vi "探头窗口-20-网络版.vi"() -> ()   [LabVIEW 2017]
panel:
  in  "外部停止命令？":bool=TRUE
  out "引用-监测模式？":refnum<vi>
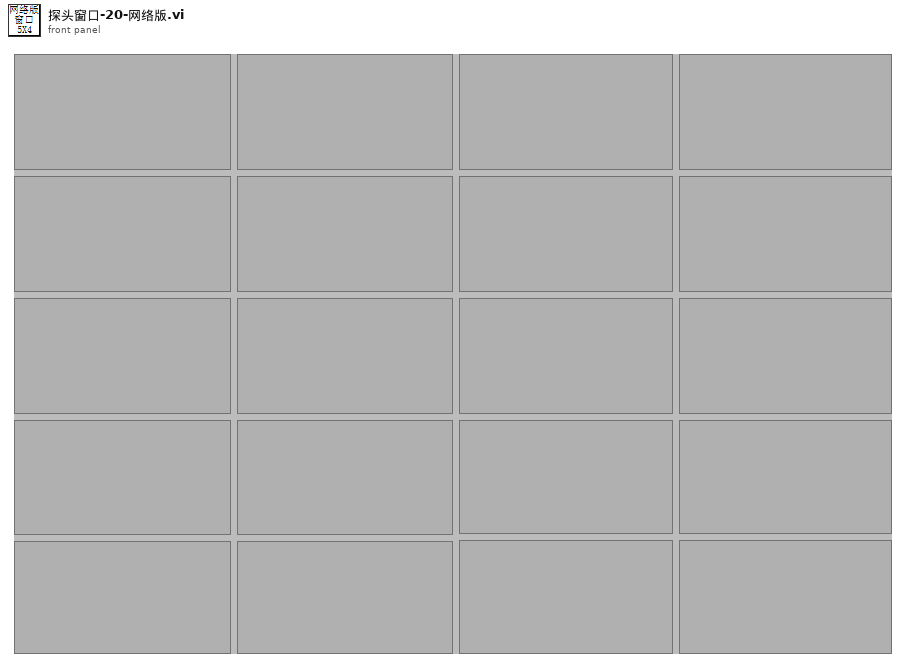
[diagram p1: front panel]
types:
  T1 = typedef "eventvkey.ctl" = enum16{"ASCII", "Enter", "Return", "Shift", "Ctrl", "Alt", "Cmd", "Opt", "Caps", "NumLock", "Clear", "Break", "Up", "Down", "Left", "Right", "Insert", "Delete", "Home", "End", "PageUp", "PageDown", "Escape", "Help", "Pause", "ScrollLock", "F1", "F2", "F3", "F4", "F5", "F6", "F7", "F8", "F9", "F10", "F11", "F12", "F13", "F14", "F15", "F16", "F17", "F18", "F19", "F20", "F21", "F22", "F23", "F24", "Play", "VolumeUp", "VolumeDown", "Mute", "Two Byte Char"}
  T2 = typedef "探头属性.ctl" = cluster{"探头地址与信息":T3, "测量值":T6, "限值":T7, "探头状态":T8, "累积记录":T9, "报警方式":T10}
  T3 = typedef "探测器信息.ctl" = cluster{"网络地址":string, "名称":string, "备注":string, "累积剂量":dbl, "累积限值":dbl, "硬件剂量率限值":T4, "剂量率限值1":dbl, "剂量率限值2":dbl, "报警方式":T5}
  T4 = typedef "探头剂量率限值选择.ctl" = enum16{"一级限值", "二级限值"}
  T5 = typedef "报警方式选择.ctl" = enum16{"常报警", "自动静音", "手动静音"}
  T6 = typedef "测量值.ctl" = cluster{"时间":timestamp, "数值":dbl}
  T7 = typedef "剂量率限值.ctl" = cluster{"限值1":dbl, "限值2":dbl, "探头限值":T4}
  T8 = typedef "探头状态.ctl" = enum16{"正常", "离线", "禁用", "一级报警", "二级报警", "累积报警"}
  T9 = typedef "单条累积记录.ctl" = cluster{"起始时间":timestamp, "结束时间":timestamp, "累积剂量":dbl}
  T10 = typedef "报警方式.ctl" = cluster{"报警方式":T5, "延迟计时":u16, "报警中？":bool}
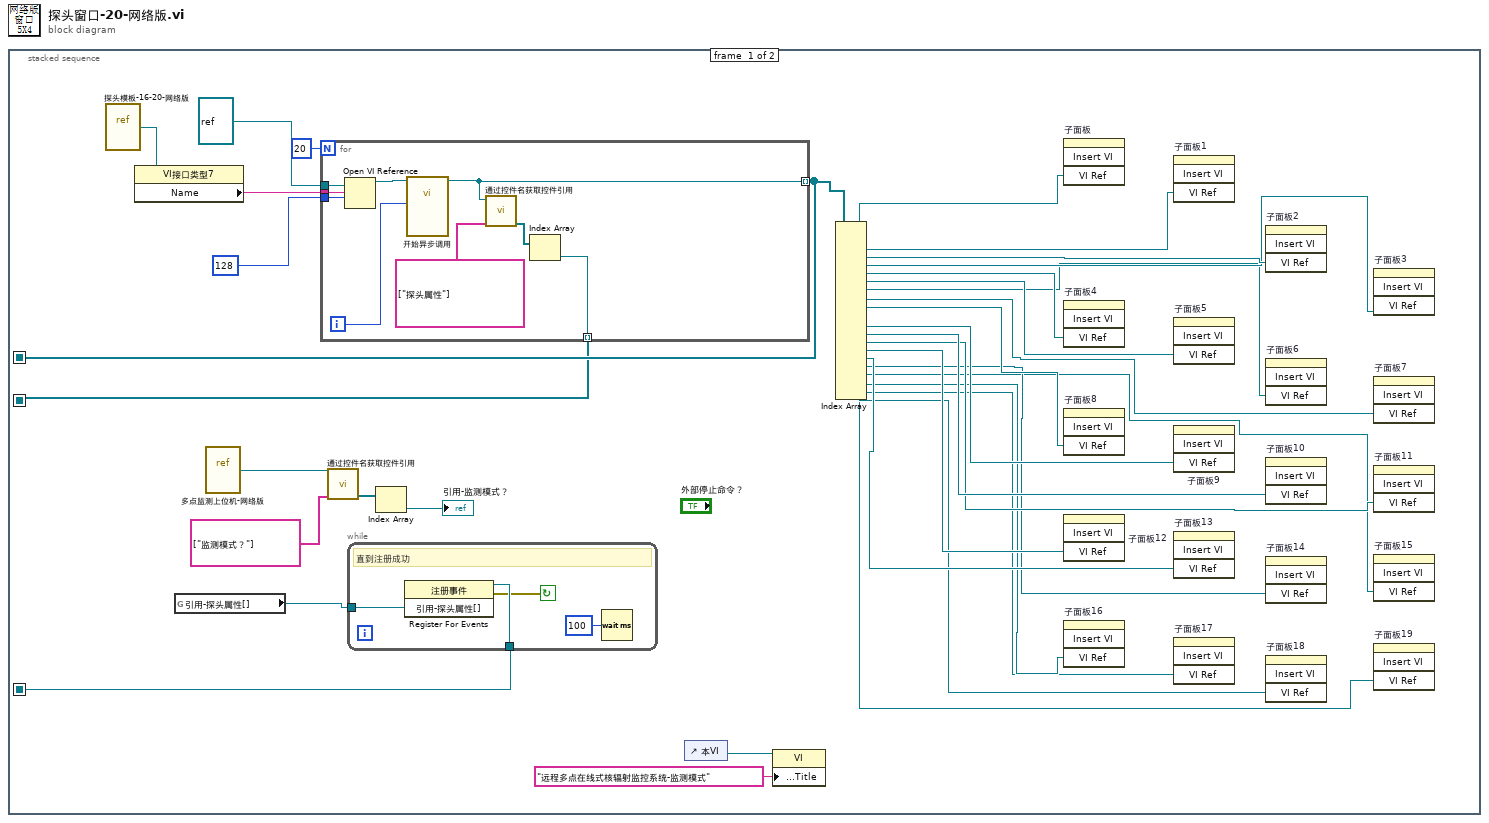
[diagram p0: block diagram]
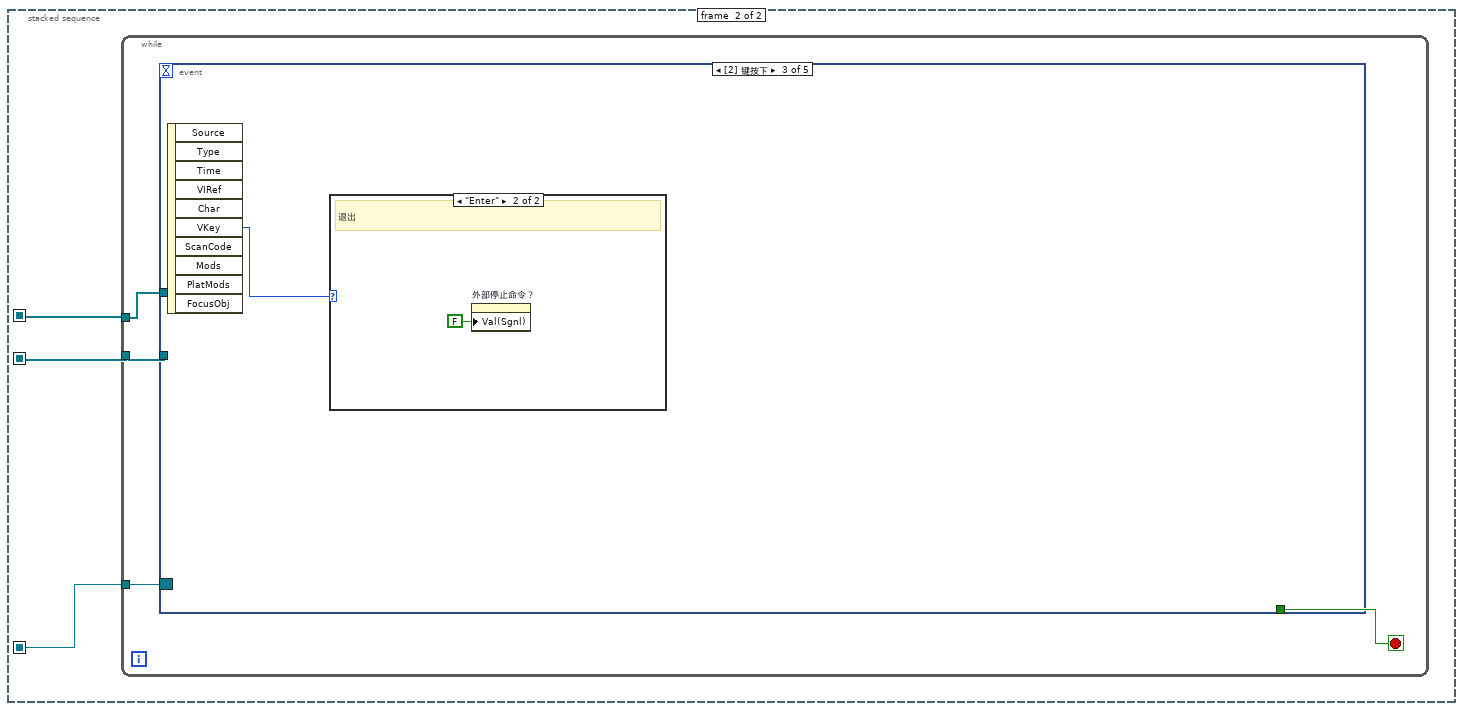
[diagram p2: hidden frame]
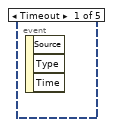
[diagram p3: hidden frame]
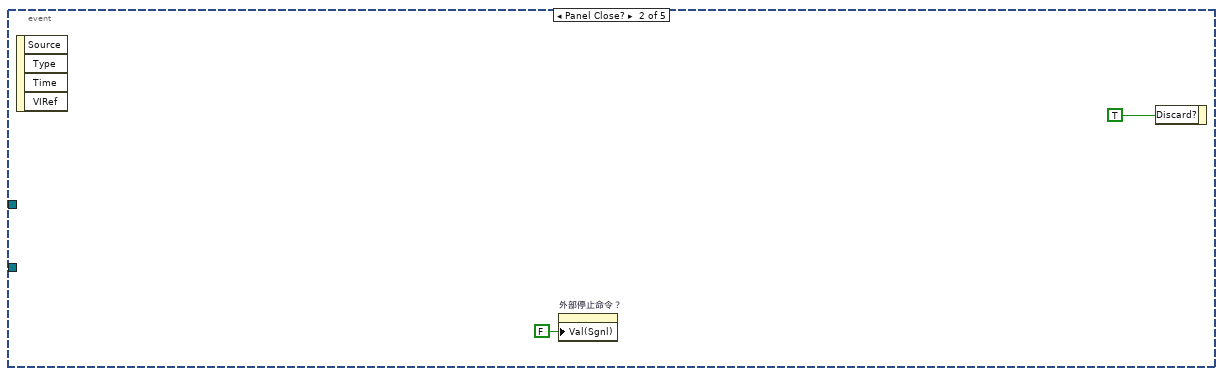
[diagram p4: hidden frame]
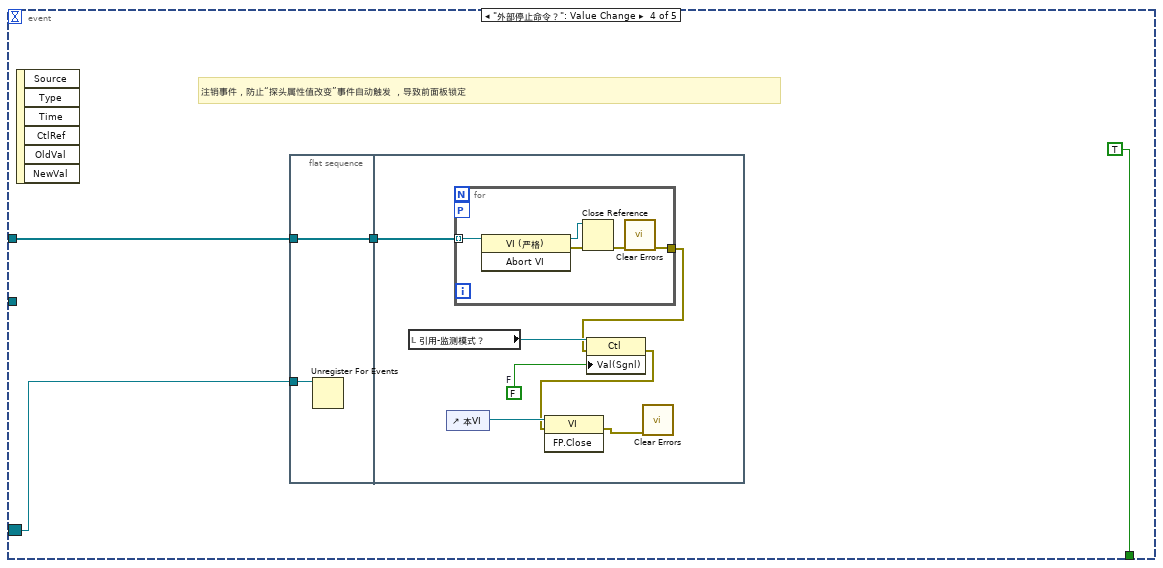
[diagram p6: hidden frame]
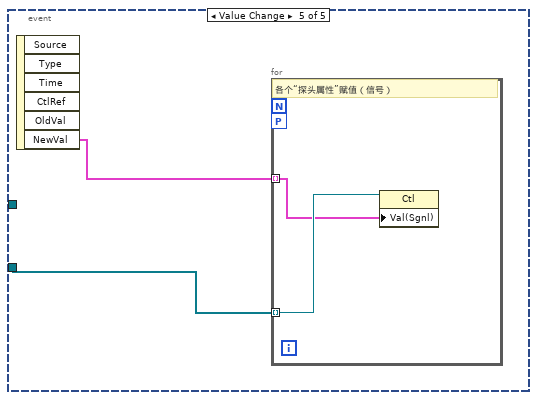
[diagram p7: hidden frame]
diagram:
  n1 = stacked-sequence {
    seq-local: [w30 _] -> [_ w51]
    seq-local: [w9 _] -> [_ w50]
    seq-local: [w1 _] -> [_ w49]
    frame #0 {
      n2 = vi-ref "探头模板-16-20-网络版.vi"() -> (w35:refnum<vi>)
      n3 = property class="VI接口类型7"(reference=w35) -> ("Name"=w34:string)  [unwired: 1 in, 2 out]
      n4 = global read "全局变量-35点监测.vi" "引用-探头属性[]"() -> (w2:refnum<vi>)
      n5 = vi-ref "多点监测上位机-网络版.vi"() -> (w5:refnum<vi>)
      n6 = for {
        N: 20 -> [_]
        tunnel: w34 -> [w48]
        tunnel: 128 ("选项") -> [w47]
        tunnel: refnum<vi> refnum ("类型说明符VI引用句柄（仅用于类型）") -> [w46]
        tunnel: [w41] -> w30 mode=indexing
        tunnel: [w42] -> w9 mode=indexing
        i -> [w40]
        n7 = Open VI Reference(type specifier VI Refnum (for type only)=w46, vi path=w48, options=w47) -> (vi reference=w43:refnum<vi>)  [unwired: 3 in, 1 out]
        n8 = call-by-ref "开始异步调用"(reference=w43, "探头序号"=w40) -> (reference out=w41:refnum<vi>)  [unwired: 12 in, 1 out]
        n9 = call "通过控件名获取控件引用.vi"("控件名数组"=string[] ["探头属性"], "VI引用"=w41) -> ("控件引用输出"=w45:refnum<vi>[])  [unwired: 7 in, 2 out]
        n10 = Index Array(array=w45) -> (element=w42:refnum<vi>)  [unwired: 1 in]
      }
      n11 = call "通过控件名获取控件引用.vi"("控件名数组"=string[] ["监测模式？"], "VI引用"=w5) -> ("控件引用输出"=w7:refnum<vi>[])  [unwired: 7 in, 2 out]
      n12 = while {
        tunnel: w2 -> [w39]
        tunnel: [w38] -> w1
        stop <- w37 continue-if-true
        # "直到注册成功"
        n13 = register-events(w39) -> (reference out=w38:refnum<event-registration>, error out=w37:errorcluster)  [unwired: 2 in]
        n14 = Wait (ms)(milliseconds to wait=u32 100 ("等待时间（毫秒）")) -> ()  [unwired: 1 out]
      }
      n15 = Index Array(array=w7) -> (element=→"引用-监测模式？":refnum<vi>)  [unwired: 1 in]
      n16 = control-ref of="本VI"() -> (w4:refnum<vi>)
      n17 = property class="VI"(reference=w4, "Front Panel.Title"="远程多点在线式核辐射监控系统-监测模式" ("前面板窗口:标题")) -> ()  [unwired: 1 in, 2 out]
      n18 = Index Array(array=w30) -> (element #1=w29:refnum<vi>, element #2=w28:refnum<vi>, element #3=w27:refnum<vi>, element #4=w26:refnum<vi>, element #5=w25:refnum<vi>, element #6=w24:refnum<vi>, element #7=w23:refnum<vi>, element #8=w22:refnum<vi>, element #9=w21:refnum<vi>, element #10=w20:refnum<vi>, element #11=w19:refnum<vi>, element #12=w18:refnum<vi>, element #13=w17:refnum<vi>, element #14=w16:refnum<vi>, element #15=w15:refnum<vi>, element #16=w14:refnum<vi>, element #17=w13:refnum<vi>, element #18=w12:refnum<vi>, element #19=w11:refnum<vi>, element #20=w10:refnum<vi>)  [unwired: 20 in]
      n19 = invoke on="子面板" class="子面板" method="Insert VI"("VI Ref"=w29) -> ()  [unwired: 3 in, 4 out]
      n20 = invoke on="子面板4" class="SubPnl" method="Insert VI"("VI Ref"=w25) -> ()  [unwired: 3 in, 4 out]
      n21 = invoke on="子面板8" class="SubPnl" method="Insert VI"("VI Ref"=w21) -> ()  [unwired: 3 in, 4 out]
      n22 = invoke on="子面板12" class="SubPnl" method="Insert VI"("VI Ref"=w17) -> ()  [unwired: 3 in, 4 out]
      n23 = invoke on="子面板16" class="SubPnl" method="Insert VI"("VI Ref"=w13) -> ()  [unwired: 3 in, 4 out]
      n24 = invoke on="子面板1" class="SubPnl" method="Insert VI"("VI Ref"=w28) -> ()  [unwired: 3 in, 4 out]
      n25 = invoke on="子面板5" class="SubPnl" method="Insert VI"("VI Ref"=w24) -> ()  [unwired: 3 in, 4 out]
      n26 = invoke on="子面板9" class="SubPnl" method="Insert VI"("VI Ref"=w20) -> ()  [unwired: 3 in, 4 out]
      n27 = invoke on="子面板13" class="SubPnl" method="Insert VI"("VI Ref"=w16) -> ()  [unwired: 3 in, 4 out]
      n28 = invoke on="子面板17" class="SubPnl" method="Insert VI"("VI Ref"=w12) -> ()  [unwired: 3 in, 4 out]
      n29 = invoke on="子面板2" class="SubPnl" method="Insert VI"("VI Ref"=w27) -> ()  [unwired: 3 in, 4 out]
      n30 = invoke on="子面板6" class="SubPnl" method="Insert VI"("VI Ref"=w23) -> ()  [unwired: 3 in, 4 out]
      n31 = invoke on="子面板10" class="SubPnl" method="Insert VI"("VI Ref"=w19) -> ()  [unwired: 3 in, 4 out]
      n32 = invoke on="子面板14" class="SubPnl" method="Insert VI"("VI Ref"=w15) -> ()  [unwired: 3 in, 4 out]
      n33 = invoke on="子面板18" class="SubPnl" method="Insert VI"("VI Ref"=w11) -> ()  [unwired: 3 in, 4 out]
      n34 = invoke on="子面板3" class="SubPnl" method="Insert VI"("VI Ref"=w26) -> ()  [unwired: 3 in, 4 out]
      n35 = invoke on="子面板7" class="SubPnl" method="Insert VI"("VI Ref"=w22) -> ()  [unwired: 3 in, 4 out]
      n36 = invoke on="子面板11" class="SubPnl" method="Insert VI"("VI Ref"=w18) -> ()  [unwired: 3 in, 4 out]
      n37 = invoke on="子面板15" class="SubPnl" method="Insert VI"("VI Ref"=w14) -> ()  [unwired: 3 in, 4 out]
      n38 = invoke on="子面板19" class="SubPnl" method="Insert VI"("VI Ref"=w10) -> ()  [unwired: 3 in, 4 out]
    }
    frame #1 {
      n39 = while {
        tunnel: w51 -> [w54]
        tunnel: w50 -> [w53]
        tunnel: w49 -> [w52]
        stop <- w55 stop-if-true
        n40 = event shown="[2] 键按下" {
          selector: w52 -> [_ _ _ w60 _]
          dyn-events: _ -> [_ _ _ _ _]
          timeout: _ -> [_ _ _ _ _]
          tunnel: [_ _ _ TRUE ("放弃？") _] -> w55
          tunnel: w54 -> [_ _ _ w62 _]
          tunnel: w53 -> [_ _ _ _ w78]
          event Timeout {
            n41 = event-data() -> ()  [unwired: 1 in, 3 out]
          }
          event Panel Close? {
            n42 = event-data() -> ()  [unwired: 1 in, 4 out]
            n43 = property on="外部停止命令？" class="Bool (严格)"("Val(Sgnl)"=FALSE ("值(信号)")) -> ()  [unwired: 2 in, 2 out]
            n44 = event-data("Discard?"=TRUE ("放弃？")) -> ()  [unwired: 1 in, 1 out]
          }
          event Key Down {
            n45 = event-data() -> ("VKey"=w58:T1)  [unwired: 1 in, 9 out]
            n46 = case shown="\"Enter\"" w58 {
              frame "ASCII", Default {
              }
              frame "Enter" {
                # "退出"
                n47 = property on="外部停止命令？" class="Bool (严格)"("Val(Sgnl)"=FALSE ("值(信号)")) -> ()  [unwired: 2 in, 2 out]
              }
            }
          }
          event "外部停止命令？": Value Change {
            # "注销事件，防止“探头属性值改变”事件自动触发 ，导致前面板锁定"
            n48 = event-data() -> ()  [unwired: 1 in, 6 out]
            n49 = flat-sequence {
              tunnel: w62 -> [w65]
              tunnel: [w65] -> w61
              tunnel: w60 -> [w64]
              tunnel: w61 -> [w72]
              frame #0 {
                n50 = Unregister For Events(event registration refnum=w64) -> ()  [unwired: 1 in, 1 out]
              }
              frame #1 {
                w71 = FALSE  # F
                n51 = local read "引用-监测模式？"() -> (w70:refnum<vi>)
                n52 = control-ref of="本VI"() -> (w69:refnum<vi>)
                n53 = for {
                  tunnel: w72 -> [w77] mode=indexing
                  workers-P: _ -> [_]
                  tunnel: [w73] -> w68
                  n54 = invoke class="VI (严格)" method="Abort VI"(reference=w77) -> (reference out=w75:refnum<vi>, error out=w76:errorcluster)  [unwired: 2 in, 1 out]
                  n55 = Close Reference(reference=w75, error in (no error)=w76) -> (error out=w74:errorcluster)
                  n56 = call <vilib>:"Clear Errors.vi"("error in (no error)"=w74) -> ("error out"=w73:errorcluster)  [unwired: 5 in, 1 out]
                }
                n57 = property class="Ctl"(reference=w70, error in=w68, "Val(Sgnl)"=w71) -> (error out=w67:errorcluster)  [unwired: 1 out]
                n58 = invoke class="VI" method="FP.Close"(reference=w69, error in=w67) -> (error out=w66:errorcluster)  [unwired: 1 in, 2 out]
                n59 = call <vilib>:"Clear Errors.vi"("error in (no error)"=w66) -> ()  [unwired: 5 in, 2 out]
              }
            }
          }
          event Value Change {
            n60 = event-data() -> ("NewVal"=w79:T2[])  [unwired: 1 in, 5 out]
            n61 = for {
              workers-P: _ -> [_]
              tunnel: w78 -> [w81] mode=indexing
              tunnel: w79 -> [w80] mode=indexing
              # "各个“探头属性”赋值（信号）"
              n62 = property class="Ctl"(reference=w81, "Val(Sgnl)"=w80) -> ()  [unwired: 1 in, 2 out]
            }
          }
        }
      }
    }
  }
